vi "Acquire.vi"(10 "Controls Ref Array":refnum<vi>[](array[refnum]), 11 "VISA resource name":refnum<visa-resource-name>) -> (0 "error out":errorcluster, 3 "VISA resource name out":refnum<visa-resource-name>)   [LabVIEW 2013]
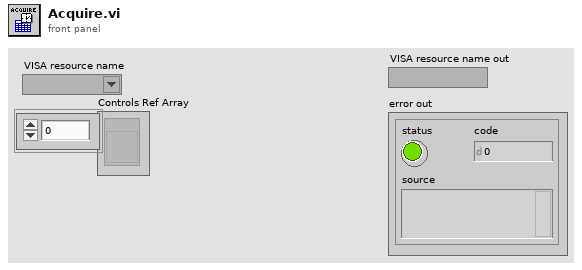
[diagram p1: front panel]
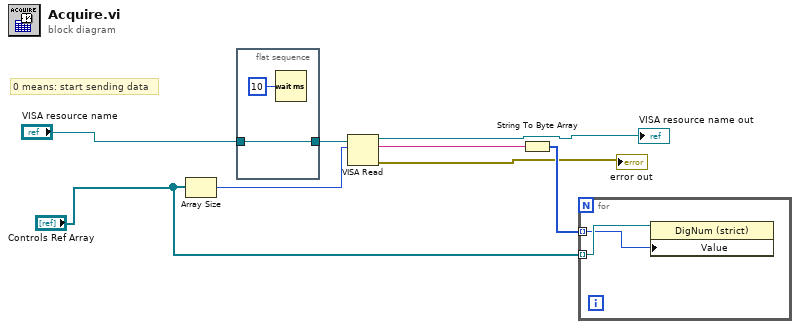
[diagram p0: block diagram]
diagram:
  # "0 means: start sending data"
  n1 = Array Size(array="Controls Ref Array") -> (size(s)=w7:i32)
  n2 = flat-sequence {
    tunnel: "VISA resource name" -> [w9]
    tunnel: [w9] -> w2
    frame #0 {
      n3 = Wait (ms)(milliseconds to wait=u32 10) -> ()  [unwired: 1 out]
    }
  }
  n4 = VISA Read(VISA resource name=w2, byte count=w7) -> (VISA resource name out=→"VISA resource name out":refnum<visa-resource-name>, read buffer=w8:string, error out=→"error out":errorcluster)  [unwired: 1 in, 1 out]
  n5 = String To Byte Array(string=w8) -> (unsigned byte array=w6:u8[])
  n6 = for {
    tunnel: w6 -> [w11] mode=indexing
    tunnel: "Controls Ref Array" -> [w12] mode=indexing
    n7 = property class="DigNum (strict)"(reference=w12, "Value"=w11) -> ()  [unwired: 1 in, 2 out]
  }
